vi "Get Type.vi"(11 "Double in":refnum<class "Double.lvclass">) -> (3 "Type":string)   [LabVIEW 2019, in "Double.lvclass"]
uses:
  <vilib>/gpm_packages/@cs/data-type-serializer/source/Double/Double.lvclass
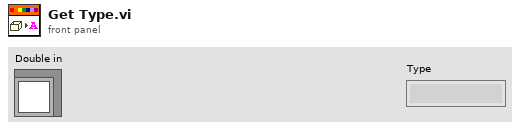
[diagram p1: front panel]
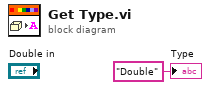
[diagram p0: block diagram]
diagram:
  "Type" <- "Double" ("Type")
